vi "event_interface_undefer_panel_updates.vi"(6 "local_interface":refnum<user-event>, 8 "error in (no error)":errorcluster) -> (0 "error out":errorcluster)   [LabVIEW 2015, in "lv-interface-re.lvlib"]
uses:
  lv-interface-re.lvlib
  _controls/event_interface.ctl
  _controls/event_interface_command.ctl
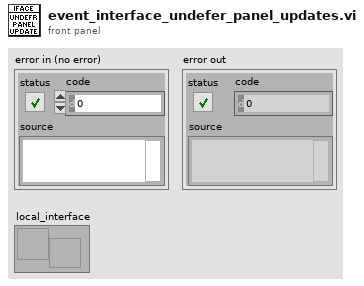
[diagram p1: front panel]
types:
  T1 = typedef "lv-interface-re.lvlib/event_interface.ctl" = cluster{"command":T2, "data":variant}
  T2 = typedef "lv-interface-re.lvlib/event_interface_command.ctl" = enum16{"<event_interface_cmd>", "defer_panel_updates", "undefer_panel_updates", "<null>"}
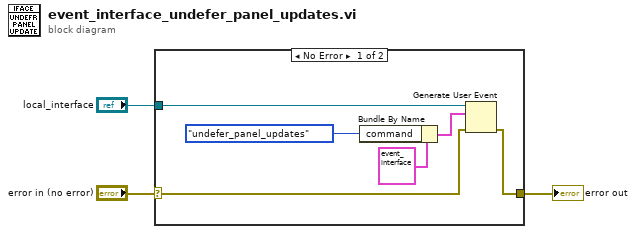
[diagram p0: block diagram]
diagram:
  n1 = case shown="No Error" "error in (no error)" {
    selector: "error in (no error)" -> [w4 w10]
    tunnel: [w9 w10] -> w3
    tunnel: "local_interface" -> [w5 _]
    frame No Error {
      n2 = Bundle By Name(cluster=T1 {"command"=enum."<event_interface_cmd>", "data"=variant}, "command"=event_interface_command."undefer_panel_updates") -> (w8:T1)
      n3 = Generate User Event(user event=w5, event data cluster=w8, error in=w4) -> (error out=w9:errorcluster)  [unwired: 1 in, 1 out]
    }
    frame Error {
    }
  }
  "error out" <- w3
